vi "Configure Channel (AIDI Scale).vi"(0 "VISA resource name":refnum<visa-resource-name>, 1 "Scaling":T1={"Floating point position (2)"=2, "Lower Scaling (0)"=0.0, "Upper Scaling (100.00)"=100.0, "Unit Character (\"\")"=""} {"Upper Scaling (100.00)" format="%_6g"; "Lower Scaling (0)" format="%_6g"; "Floating point position (2)" min=0 max=5 step=1}, 5 "Channel (0001)":string="0001", 7 "Enable Channel (True)":bool=TRUE, 9 "Span":T2={"DI Type (0: LVL)"=0, "Lower Span (0)"=0, "Upper Span (1)"=1} {"DI Type (0: LVL)" items=["LVL", "DI"]; "Upper Span (1)" min=-99999 max=99999 step=1; "Lower Span (0)" min=-99999 max=99999 step=1}, 11 "error in (no error)":errorcluster) -> (4 "VISA resource name out":refnum<visa-resource-name>, 6 "Channel":string, 15 "error out":errorcluster)   [LabVIEW 2020, in "Yokogawa GX Series.lvlib"]
doc: "Sets the input range as Contact.\n\nCommand: SRangeAI"
uses:
  <instrlib>/Yokogawa GX Series/Yokogawa GX Series.lvlib
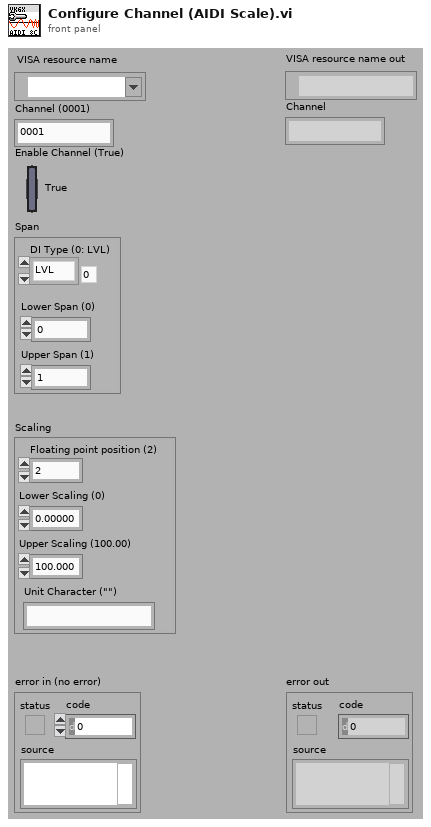
[diagram p1: front panel]
types:
  T1 = cluster{"Floating point position (2)":i32, "Lower Scaling (0)":dbl, "Upper Scaling (100.00)":dbl, "Unit Character (\"\")":string}
  T2 = cluster{"DI Type (0: LVL)":i32, "Lower Span (0)":i32, "Upper Span (1)":i32}
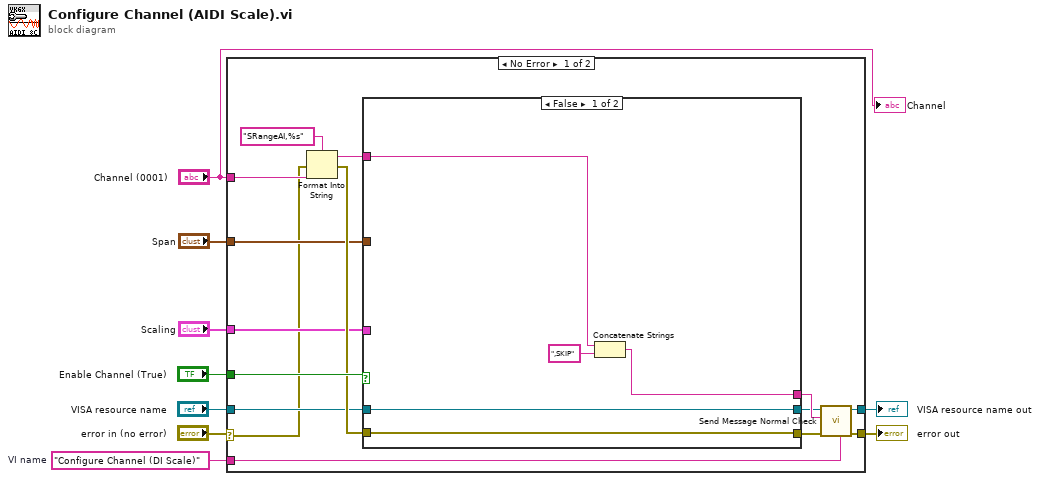
[diagram p0: block diagram]
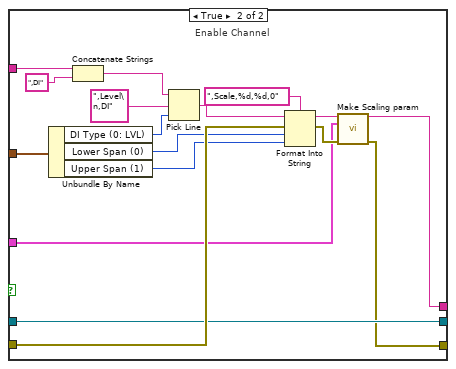
[diagram p2: hidden frame]
diagram:
  w9 = "Configure Channel (DI Scale)"  # VI name
  n1 = case shown="No Error" "error in (no error)" {
    selector: "error in (no error)" -> [w10 w47]
    tunnel: w9 -> [w23 _]
    tunnel: "Enable Channel (True)" -> [w21 _]
    tunnel: [w20 w48] -> w7
    tunnel: [w19 w47] -> w6
    tunnel: "Span" -> [w16 _]
    tunnel: "VISA resource name" -> [w15 w48]
    tunnel: "Scaling" -> [w12 _]
    tunnel: "Channel (0001)" -> [w11 _]
    frame No Error {
      n2 = Format Into String(format string="SRangeAI,%s", error in=w10, w11) -> (resulting string=w18:string, error out=w17:errorcluster)  [unwired: 1 in]
      n3 = case shown="False" w21 {
        tunnel: w18 -> [w27 w42]
        tunnel: [w26 w30] -> w13
        tunnel: [w28 w31] -> w22
        tunnel: w17 -> [w26 w45]
        tunnel: w16 -> [_ w44]
        tunnel: w12 -> [_ w32]
        tunnel: [w25 w35] -> w14
        tunnel: w15 -> [w25 w35]
        frame False {
          n4 = Concatenate Strings(w27, ",SKIP") -> (w28:string)
        }
        frame True {
          # "Enable Channel"
          n5 = Unbundle By Name(w44) -> ("DI Type (0: LVL)"=w40:i32, "Lower Span (0)"=w37:i32, "Upper Span (1)"=w36:i32)
          n6 = Concatenate Strings(w42, ",DI") -> (w39:string)
          n7 = Pick Line(string ("")=w39, multi-line string=",Level\n,DI", line index=w40) -> (output string=w38:string)
          n8 = Format Into String(format string=",Scale,%d,%d,0", initial string=w38, error in=w45, w37, w36) -> (resulting string=w34:string, error out=w33:errorcluster)
          n9 = call <instrlib>:"Make Scaling param.vi"("String (\"\")"=w34, "Scaling"=w32, "error in (no error)"=w33) -> ("String After"=w31:string, "error out"=w30:errorcluster)  [unwired: 11 in]
        }
      }
      n10 = call <instrlib>:"Send Message Normal Check.vi"("Source (\"\")"=w23, "error in (no error)"=w13, "Send Message (\"\")"=w22, "VISA resource name"=w14) -> ("error out"=w19:errorcluster, "VISA resource name out"=w20:refnum<visa-resource-name>)  [unwired: 2 in, 4 out]
    }
    frame Error {
    }
  }
  "error out" <- w6
  "VISA resource name out" <- w7
  "Channel" <- "Channel (0001)"
